vi "UI.vi"() -> ()   [LabVIEW 2020]
panel:
  in  "Btn_ Send _Caller":bool
  out "Message_cpt":u8
  in  "Btn_Error":bool
  in  "Btn_Launch":bool
  in  "Message":string
  out "Display":string
  in  "Btn_ Send":bool
  in  "Btn_Error":bool
  out "Waveform Chart":dbl(graph)
  out "Message":u8
  in  "Btn_PopController":bool
  in  "Btn_ popCaller":bool
  in  "Btn_Error":bool
  in  "Btn_Launch":bool
  in  "Message":string
  out "Display":string
  in  "Btn_ Send":bool
  in  "Btn_Error":bool
  in  "Btn_Error":bool
  in  "Btn_Launch":bool
  in  "Message":string
  out "Display":string
  in  "Btn_ Send 2":bool
  # "Nested"
  # "Caller"
  # "Caller"
  # "Nested"
  # "Nested"
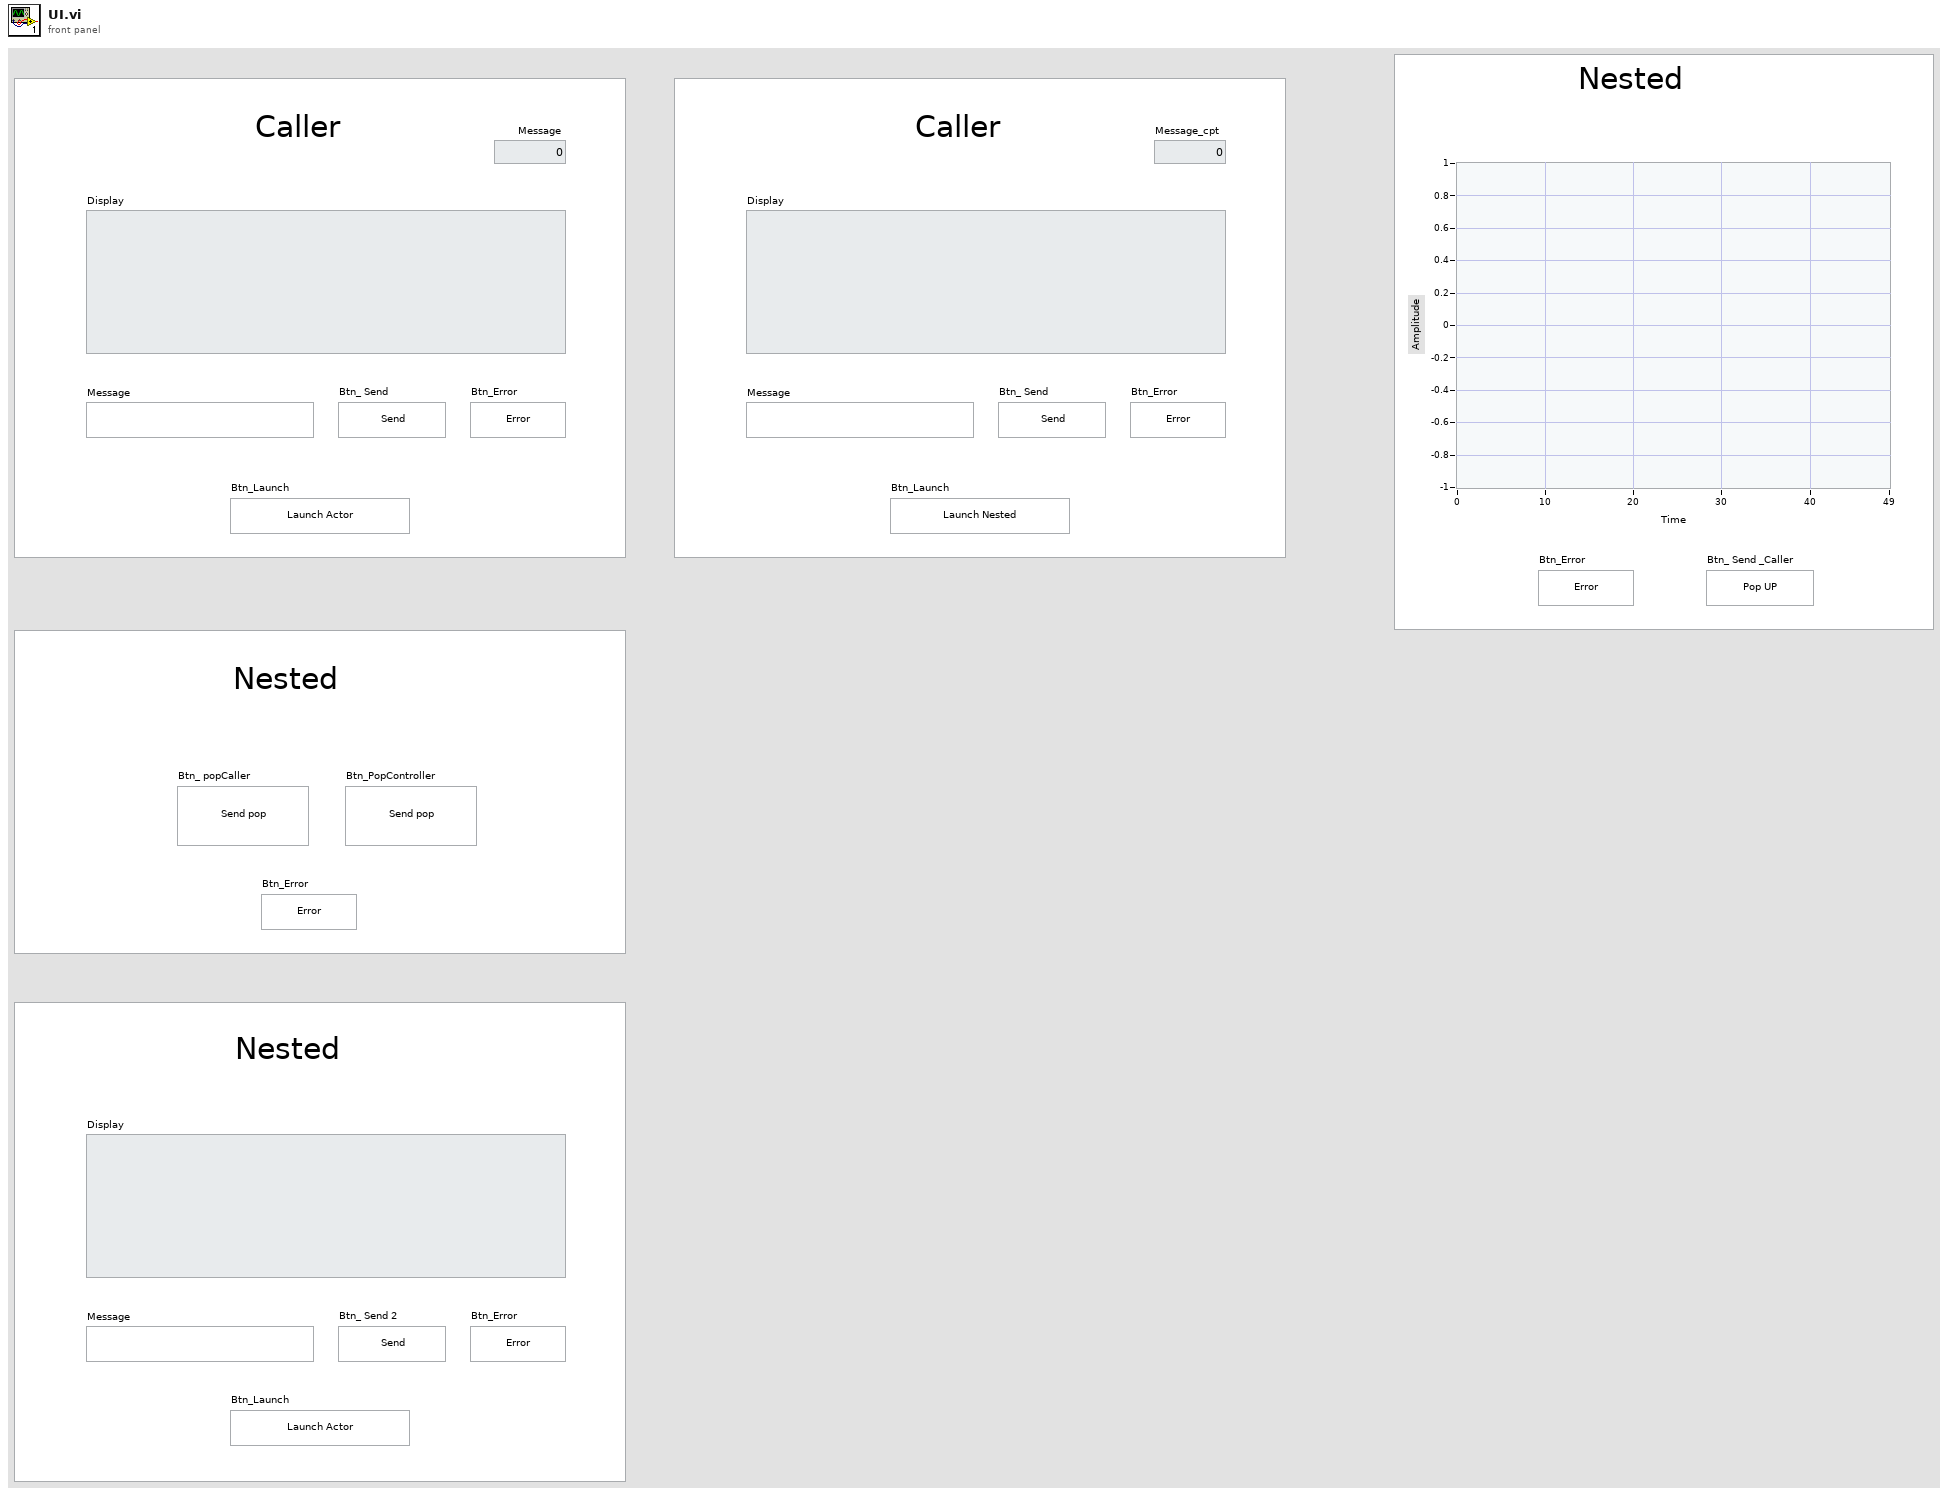
[diagram p1: front panel]
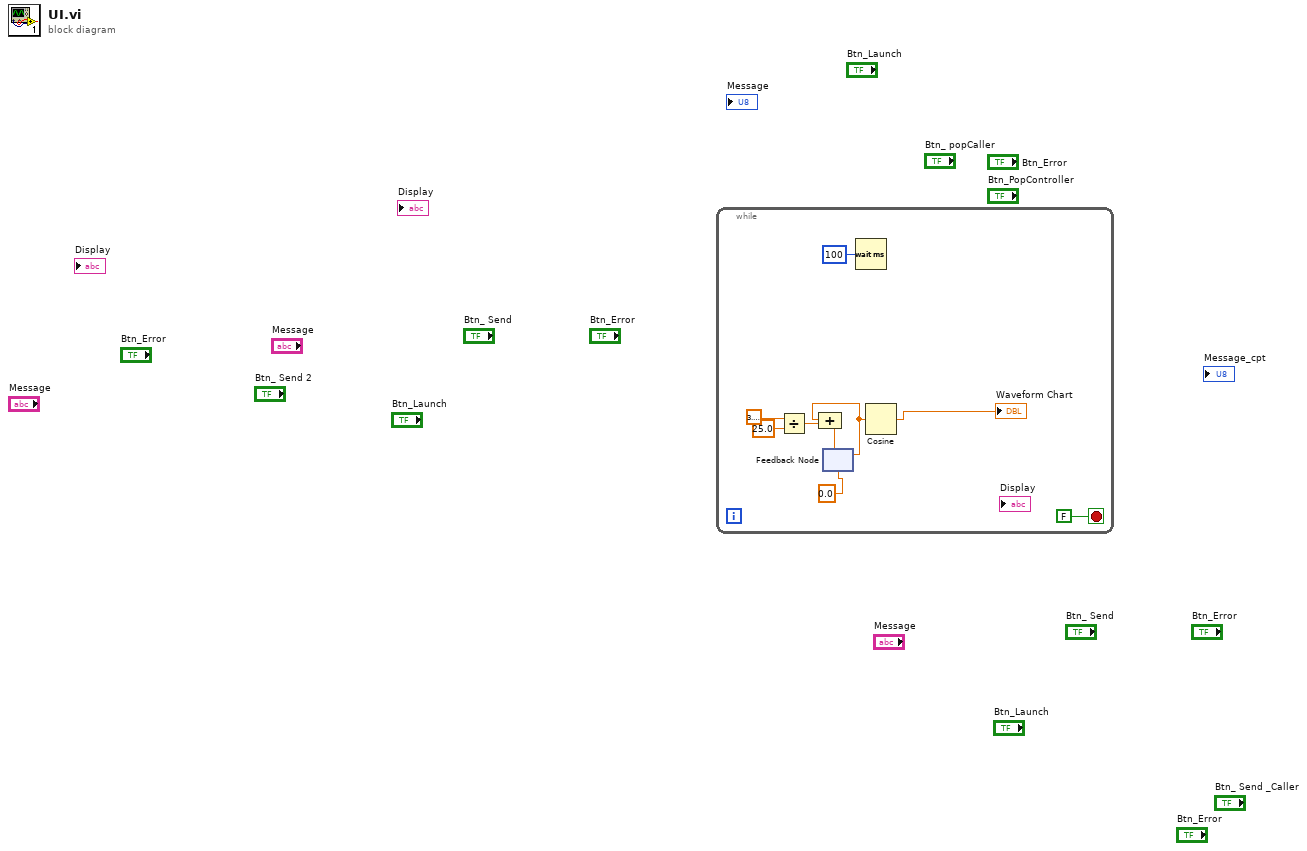
[diagram p0: block diagram]
diagram:
  n1 = while {
    stop <- FALSE stop-if-true
    n2 = Divide(x=3.141592653589793, y=25.0) -> (x/y=w7:dbl)
    n3 = feedback #1(0.0) -> (w3:dbl)
    n4 = Compound Arithmetic op=ADD(w3, w7) -> (w4:dbl)
    n5 = feedback-in #1(w4) -> ()
    n6 = Wait (ms)(milliseconds to wait=u32 100) -> ()  [unwired: 1 out]
    n7 = Cosine(x=w3) -> (cos(x)=→"Waveform Chart":dbl)
  }
